vi "Abort.vi"(8 "error in":errorcluster, 9 "H/C state":dbl, 10 "stop":bool) -> (0 "error in 2":errorcluster)   [LabVIEW 2015]
uses:
  TC/heating or cooling.vi
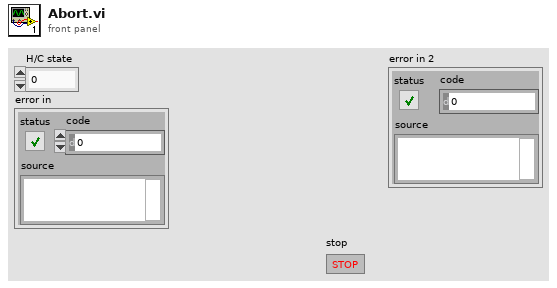
[diagram p1: front panel]
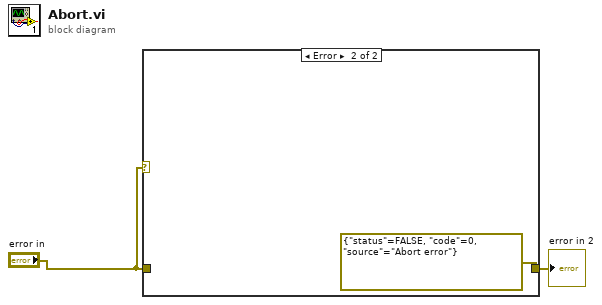
[diagram p0: block diagram]
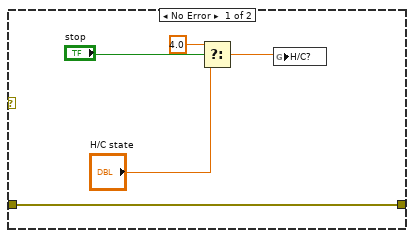
[diagram p2: hidden frame]
diagram:
  n1 = case shown="Error" "error in" {
    tunnel: "error in" -> [w3 _]
    tunnel: [w3 errorcluster {"status"=FALSE, "code"=0, "source"="Abort error"} ("error in")] -> w2
    frame No Error {
      n2 = Select(t=4.0, s="stop", f="H/C state") -> (s? t:f=w6:dbl)
      n3 = global write "heating or cooling.vi" "H/C?"(w6) -> ()
    }
    frame Error {
    }
  }
  "error in 2" <- w2
